vi "SpeedID.vi"(10 "String":string, 11 "Speed In":dbl format="%#_13g") -> (3 "Speed Out":dbl)   [LabVIEW 2016]
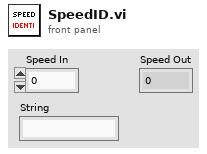
[diagram p1: front panel]
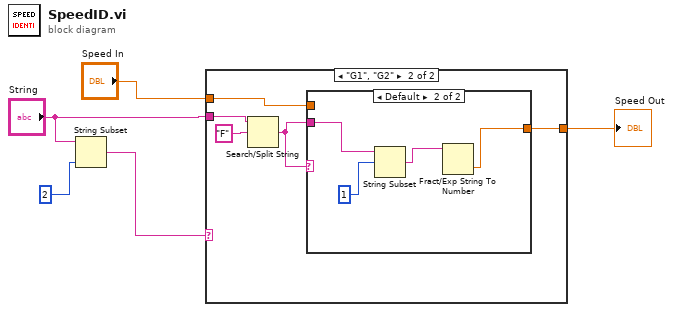
[diagram p0: block diagram]
diagram:
  n1 = String Subset(string="String", length (rest)=2) -> (substring=w4:string)  [unwired: 1 in]
  n2 = case shown="\"G1\", \"G2\"" w4 {
    tunnel: "String" -> [_ w11]
    tunnel: "Speed In" -> [w6 w8]
    tunnel: [w6 w7] -> w1
    frame Default {
    }
    frame "G1", "G2" {
      n3 = Search/Split String(string=w11, search string/char (-)="F") -> (match + rest of string=w9:string)  [unwired: 1 in, 2 out]
      n4 = case shown="Default" w9 {
        tunnel: w9 -> [_ w16]
        tunnel: w8 -> [w12 _]
        tunnel: [w12 w13] -> w7
        frame "\u0000" {
        }
        frame Default {
          n5 = String Subset(string=w16, offset (0)=1) -> (substring=w14:string)  [unwired: 1 in]
          n6 = Fract/Exp String To Number(string=w14) -> (number=w13:dbl)  [unwired: 3 in, 1 out]
        }
      }
    }
  }
  "Speed Out" <- w1
